vi "MergeByte.vi"(1 "Offset":fxp<+/-,32,16>, 2 "Resolution":fxp<+/-,32,16>, 3 "HighByte":u8, 4 "LowByte":u8) -> (0 "Result":fxp<+/-,32,16>)   [LabVIEW 2013]
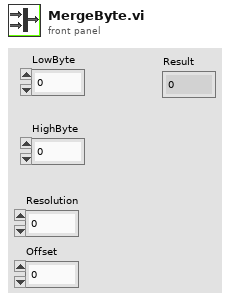
[diagram p1: front panel]
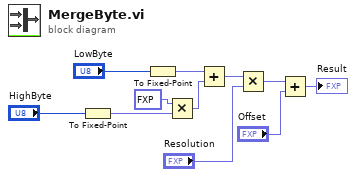
[diagram p0: block diagram]
diagram:
  n1 = To Fixed-Point(number="HighByte") -> (fixed-point=w1:fxp<+,8,8>)  [unwired: 1 in]
  n2 = To Fixed-Point(number="LowByte") -> (fixed-point=w3:fxp<+,8,8>)  [unwired: 1 in]
  n3 = Multiply(x=fxp<+,1,9> 256.0, y=w1) -> (x*y=w11:fxp<+,8,16>)
  n4 = Add(x=w3, y=w11) -> (x+y=w10:fxp<+,16,16>)
  n5 = Multiply(x=w10, y="Resolution") -> (x*y=w8:fxp<+/-,48,32>)
  n6 = Add(x=w8, y="Offset") -> (x+y=→"Result":fxp<+/-,48,32>)
